vi "Example of an Array of XY Arrays.vi"() -> ()   [LabVIEW 2011]
doc: "Example of an array of clusters of X and Y arrays of DBLs, to and from JSON using the Variant JSON tools."
uses:
  vi.lib/Addons/JSON API/JSON Value/Get as JSON string.vi
  vi.lib/Addons/JSON API/JSON Value/Set from JSON string.vi
  vi.lib/Addons/JSON API/Variant JSON/Variant to JSON.vi
  vi.lib/Addons/JSON API/Variant JSON/Get as Variant.vi
  vi.lib/Addons/JSON API/JSON Value/Get Item by name array.vi
  vi.lib/Addons/JSON API/JSON Value/JSON Value.lvclass
  vi.lib/Addons/JSON API/Get Polymorphic/JSON GetSet.lvlib
  vi.lib/Addons/JSON API/Variant JSON/Variant JSON.lvlib
panel:
  out "JSON string length":i32 format="%_3p"
  out "Total number of DBL Values":i32
  out "To Variant":dbl format="%#_3p"
  out "from JSON":dbl format="%#_3p"
  out "To JSON":dbl format="%#_3p"
  out "Set Variant":dbl format="%#_3p"
  out "XY Graph":cluster{"X":dbl[], "Y":dbl[]}[](graph)
  in  "Number of XY plots":i32=10
  in  "Number of readings per XY plot":i32=1000
  # "Example of an array of clusters of X and Y arrays of DBLs, to and from JSON using the Variant JSON tools."
  # "Times, divided by total number of DBL values"
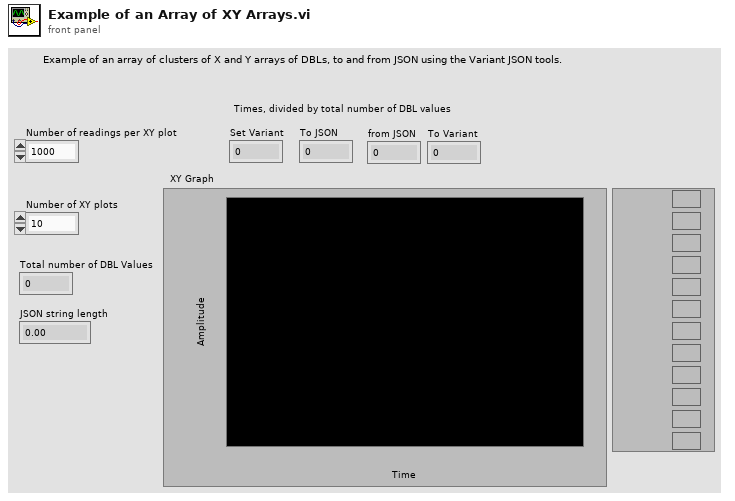
[diagram p1: front panel]
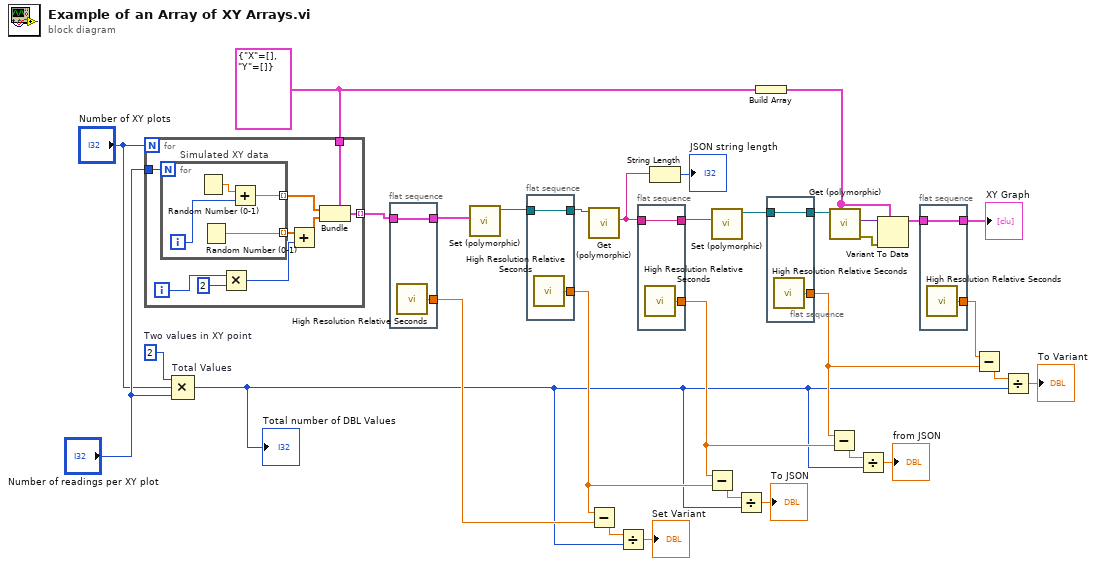
[diagram p0: block diagram]
diagram:
  w16 = 2  # Two values in XY point
  w30 = cluster{"X":dbl[], "Y":dbl[]} {"X"=[], "Y"=[]} ("cluster")
  n1 = for {
    N: "Number of XY plots" -> [_]
    tunnel: [w39] -> w28 mode=indexing
    tunnel: "Number of readings per XY plot" -> [w38]
    tunnel: w30 -> [w37]
    i -> [w35]
    n2 = for "Simulated XY data" {
      N: w38 -> [_]
      tunnel: [w43] -> w40 mode=indexing
      tunnel: [w42] -> w41 mode=indexing
      i -> [w44]
      n3 = Random Number (0-1)() -> (number: 0 to 1=w45:dbl)
      n4 = Random Number (0-1)() -> (number: 0 to 1=w43:dbl)
      n5 = Add(x=w45, y=w44) -> (x+y=w42:dbl)
    }
    n6 = Multiply(x=w35, y=2) -> (x*y=w33:i32)
    n7 = Add(x=w40, y=w33) -> (x+y=w36:dbl[])
    n8 = Bundle(cluster=w37, "X"=w41, "Y"=w36) -> (w39:cluster{"X":dbl[], "Y":dbl[]})
  }
  n9 = Compound Arithmetic op=MULTIPLY "Total Values"(w16, "Number of XY plots", "Number of readings per XY plot") -> (w3:i32)
  "Total number of DBL Values" <- w3
  n10 = flat-sequence {
    tunnel: [w47] -> w27
    tunnel: w28 -> [w47]
    tunnel: [w46] -> w19
    frame #0 {
      n11 = call <vilib>:"High Resolution Relative Seconds.vi"() -> ("relative seconds"=w46:dbl)
    }
  }
  n12 = call-poly "Set (polymorphic).vi"("Variant"=w27) -> ("JSON Value out"=w25:refnum<class "JSON Value.lvclass">)  [unwired: 9 in, 1 out]
  n13 = flat-sequence {
    tunnel: [w49] -> w26
    tunnel: w25 -> [w49]
    tunnel: [w48] -> w11
    frame #0 {
      n14 = call <vilib>:"High Resolution Relative Seconds.vi"() -> ("relative seconds"=w48:dbl)
    }
  }
  n15 = call-poly "Get (polymorphic).vi"("JSON Value in"=w26) -> ("String"=w2:string)  [unwired: 9 in, 1 out]
  n16 = Subtract(x=w11, y=w19) -> (x-y=w15:dbl)
  n17 = Divide(x=w15, y=w3) -> (x/y=→"Set Variant":dbl)
  n18 = flat-sequence {
    tunnel: [w51] -> w24
    tunnel: w2 -> [w51]
    tunnel: [w50] -> w8
    frame #0 {
      n19 = call <vilib>:"High Resolution Relative Seconds.vi"() -> ("relative seconds"=w50:dbl)
    }
  }
  n20 = String Length(string=w2) -> (length=→"JSON string length":i32)
  n21 = Subtract(x=w8, y=w11) -> (x-y=w12:dbl)
  n22 = call-poly "Set (polymorphic).vi"("JSON stream"=w24) -> ("JSON Value out"=w23:refnum<class "JSON Value.lvclass">)  [unwired: 8 in, 2 out]
  n23 = Divide(x=w12, y=w3) -> (x/y=→"To JSON":dbl)
  n24 = Build Array(w30) -> (w29:cluster{"X":dbl[], "Y":dbl[]}[])
  n25 = flat-sequence {
    tunnel: [w53] -> w22
    tunnel: w23 -> [w53]
    tunnel: [w52] -> w4
    frame #0 {
      n26 = call <vilib>:"High Resolution Relative Seconds.vi"() -> ("relative seconds"=w52:dbl)
    }
  }
  n27 = Subtract(x=w4, y=w8) -> (x-y=w10:dbl)
  n28 = call-poly "Get (polymorphic).vi"("Variant (Data Type)"=w29, "JSON in"=w22) -> ("error out"=w32:errorcluster, "Variant out"=w31:variant)  [unwired: 7 in, 1 out]
  n29 = Divide(x=w10, y=w3) -> (x/y=→"from JSON":dbl)
  n30 = Variant To Data(error in=w32, type=w29, Variant=w31) -> (data=w21:cluster{"X":dbl[], "Y":dbl[]}[])  [unwired: 1 out]
  n31 = flat-sequence {
    tunnel: [w55] -> w20
    tunnel: w21 -> [w55]
    tunnel: [w54] -> w5
    frame #0 {
      n32 = call <vilib>:"High Resolution Relative Seconds.vi"() -> ("relative seconds"=w54:dbl)
    }
  }
  n33 = Subtract(x=w5, y=w4) -> (x-y=w6:dbl)
  n34 = Divide(x=w6, y=w3) -> (x/y=→"To Variant":dbl)
  "XY Graph" <- w20
